vi "4.4.vi"() -> ()   [LabVIEW 2017]
panel:
  in  "数值":dbl
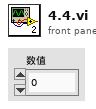
[diagram p1: front panel]
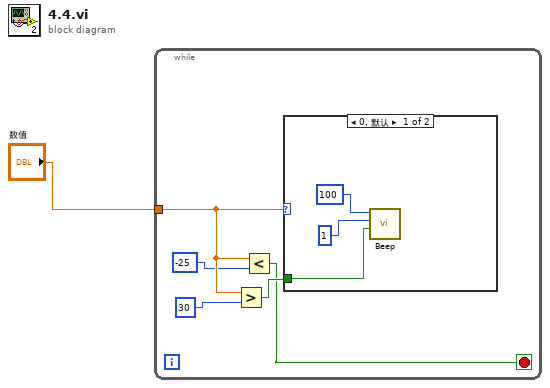
[diagram p0: block diagram]
diagram:
  n1 = while {
    tunnel: "数值" -> [w6]
    stop <- w2 stop-if-true
    n2 = Greater?(x=w6, y=30) -> (0:w3:bool)
    n3 = Less?(x=w6, y=-25) -> (x < y?=w2:bool)
    n4 = case shown="0, 默认" w6 {
      tunnel: w3 -> [w9 _]
      frame 0, Default {
        n5 = call <vilib>:"Beep.vi"("use system alert? (T)"=w9, "duration (msec)"=1, "frequency (Hz)"=100) -> ()  [unwired: 9 in]
      }
      frame 1 {
      }
    }
  }
